vi "sortRobotsFeedback.vi"(8 "error in (no error)":errorcluster, 11 "robotsFeedback in":cluster{"id":u32, "dribblerContact":bool}[](array[cluster])) -> (0 "error out":errorcluster, 3 "robotsFeedback out":cluster{"id":u32, "dribblerContact":bool}[](array[cluster]))   [LabVIEW 2020, in "Communication.lvclass"]
uses:
  Communication.lvclass
panel:
  out "Communication out":refnum<class "Communication.lvclass">
  in  "Communication in":refnum<class "Communication.lvclass">
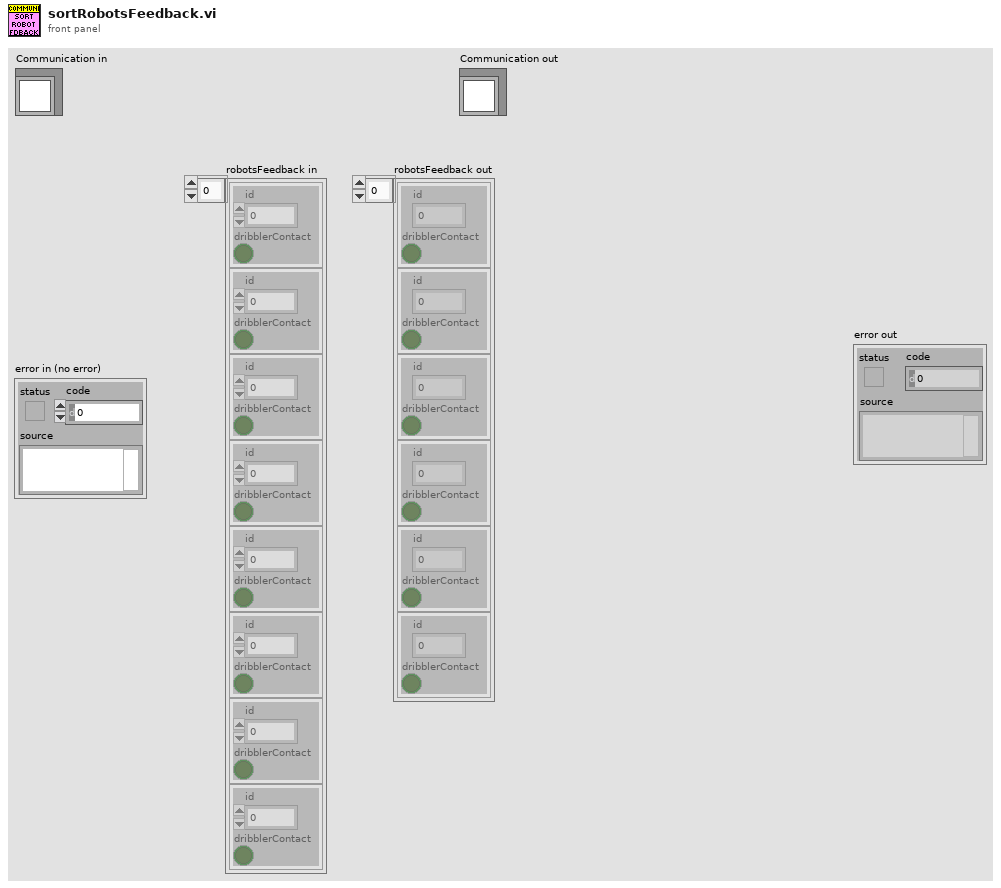
[diagram p1: front panel]
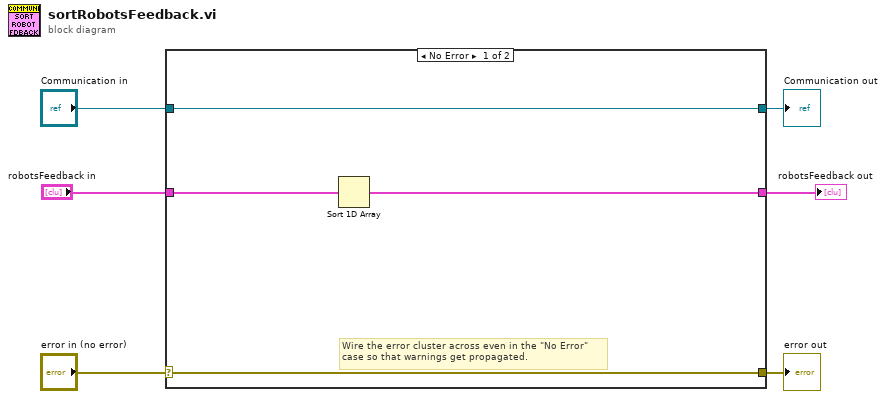
[diagram p0: block diagram]
diagram:
  n1 = case shown="No Error" "error in (no error)" {
    selector: "error in (no error)" -> [w9 w12]
    tunnel: [w9 w12] -> w5
    tunnel: [w10 w11] -> w3
    tunnel: "Communication in" -> [w10 w11]
    tunnel: "robotsFeedback in" -> [w8 _]
    tunnel: [w7 _] -> w1
    frame No Error {
      # "Wire the error cluster across even in the \"No Error\"\ncase so that warnings get propagated."
      n2 = Sort 1D Array(array=w8) -> (sorted array=w7:cluster{"id":u32, "dribblerContact":bool}[])
    }
    frame Error {
    }
  }
  "error out" <- w5
  "Communication out" <- w3
  "robotsFeedback out" <- w1
